vi "CommandMotorControl.vi"(8 "PID gains":T1={"proportional gain (Kc)"=1.0, "integral time (Ti, min)"=0.01, "derivative time (Td, min)"=0.0} {"derivative time (Td, min)" format="%.3f"; "integral time (Ti, min)" format="%.3f"; "proportional gain (Kc)" format="%.3f"}, 9 "Number of Motors":u8(ring) items=["4", "6"], 10 "height":dbl format="%.2f", 11 "commanded height":dbl min=-1.0 max=1.0) -> (3 "Motor Commands":dbl[](array[numeric]))   [LabVIEW 2017]
uses:
  <vilib>/addons/control/pid/pid.llb/PID (DBL).vi
  <vilib>/addons/control/pid/NI_PID_pid.lvlib
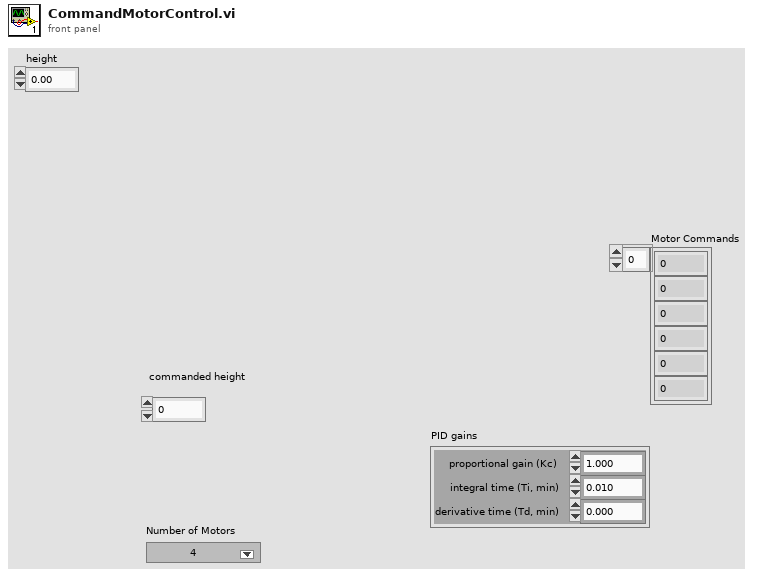
[diagram p1: front panel]
types:
  T1 = cluster{"proportional gain (Kc)":dbl, "integral time (Ti, min)":dbl, "derivative time (Td, min)":dbl}
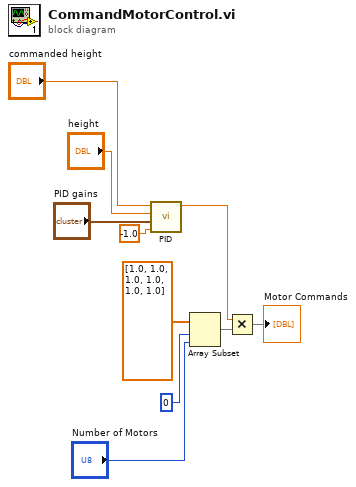
[diagram p0: block diagram]
diagram:
  n1 = call-poly <vilib>:"PID.vi"("dt (s)"=-1.0, "PID gains"="PID gains", "process variable"="height", "setpoint"="commanded height") -> ("output"=w2:dbl)  [unwired: 6 in, 1 out]
  n2 = Array Subset(array=dbl[] [1.0, 1.0, 1.0, 1.0, 1.0, 1.0], index=0, length="Number of Motors") -> (w3:dbl[])
  n3 = Multiply(x=w2, y=w3) -> (x*y=→"Motor Commands":dbl[])
